vi "Clear Display.vi"(8 "error in (no error)":errorcluster, 11 "Refnum in":T1) -> (0 "error out":errorcluster, 3 "Refnum out":T1)   [LabVIEW 2019, in "HD44780.lvlib"]
uses:
  HD44780.lvlib
  <vilib>/rvi/interface/nirviReadWriteControl/nirviReadWriteControl.xnode
  FPGA VI Reference.ctl
  NiFpgaLv.dll
  <vilib>/Utility/error.llb/Error Cluster From Error Code.vi
  <vilib>/rvi/interface/Simulation/niFpgaSimulationCallBeginRW.vi
  <vilib>/rvi/errors/niLvFpgaAdjustHostInterfaceError.vi
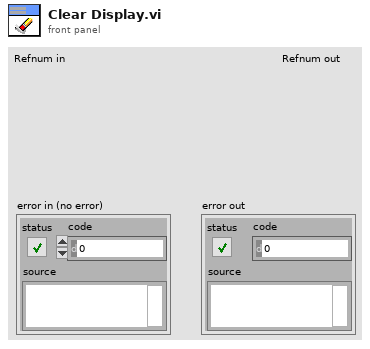
[diagram p1: front panel]
types:
  T1 = typedef "FPGA VI Reference.ctl" = refnum<k20>
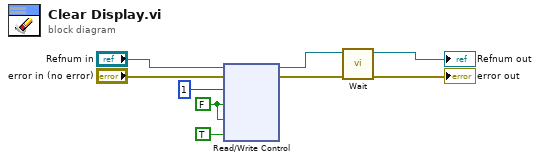
[diagram p0: block diagram]
diagram:
  w8 = FALSE ("RS")
  n1 = xnode "Read/Write Control"("FPGA VI Reference In"="Refnum in", "error in"="error in (no error)", "Data In"=u8 1, "RS"=w8, "R/W"=w8, "Enable"=TRUE) -> ("FPGA VI Reference Out"=w2:T1, "error out"=w4:errorcluster)
  n2 = call "Wait.vi"("error in (no error)"=w4, "Refnum in"=w2) -> ("error out"=→"error out":errorcluster, "Refnum out"=→"Refnum out":T1)  [unwired: 8 in]
